vi "ex_FileReadTDM.vi"(0 "file path in":path, 1 "Read specified segment size":bool, 2 "First time?":bool, 3 "Ask user for file":bool, 4 "Segment Size":i32, 5 "error in (no error)":errorcluster, 6 "Plugin info":T1, 7 "read info in":T2, 9 "single values":bool, 10 "Lock file":bool) -> (13 "read info out":T2, 14 "file path out":path, 15 "Comment":string, 16 "Signals":waveform(dbl)[](array[waveform]), 17 "Description":string, 18 "EOF":bool, 19 "error out":errorcluster)   [LabVIEW 2020]
uses:
  <vilib>/Platform/express/TDMExpress.llb/ex_readInfoTDM.ctl
  <vilib>/Platform/express/TDMExpress.llb/ex_readChannelInfo.ctl
  <vilib>/express/express shared/ExFile.llb/ex_TdmData.ctl
  <vilib>/express/express shared/ExFile.llb/ex_TdmProperty.ctl
  <vilib>/express/express shared/ex_EditUserDefinedProperties/usiDataType.ctl
  <vilib>/express/express shared/ExFile.llb/ex_PluginInfo.ctl
  <vilib>/express/express shared/ExFile.llb/ex_FileFormatSelector.ctl
  <vilib>/express/express shared/ExFile.llb/ex_FileGlobals.vi
  <vilib>/Platform/storage/Storage.llb/__closeStorageFromObject.vi
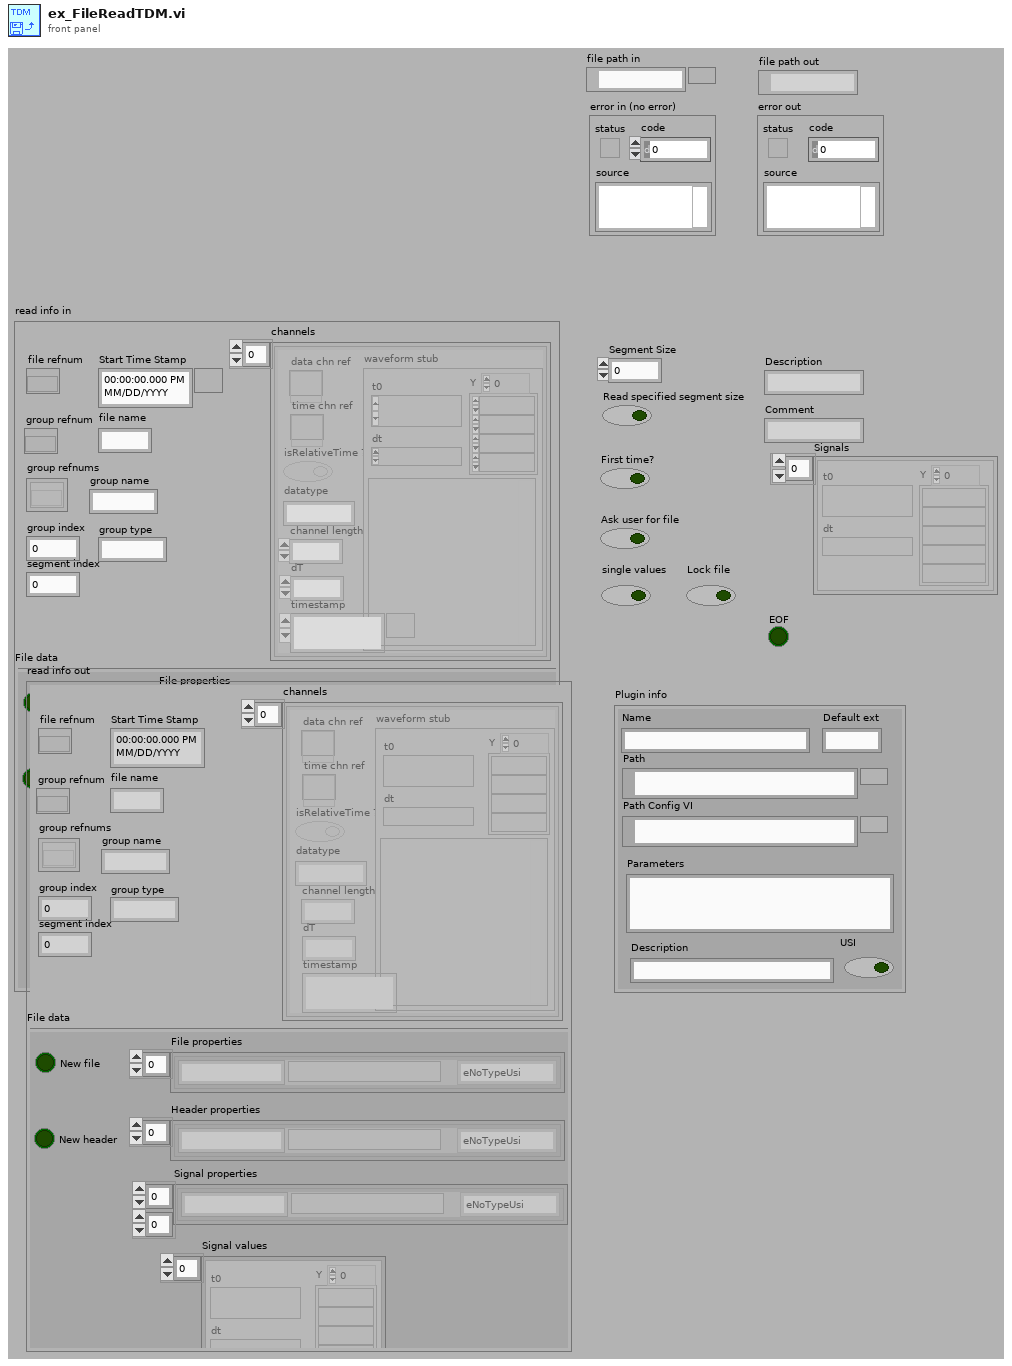
[diagram p1: front panel]
types:
  T1 = typedef "ex_PluginInfo.ctl" = cluster{"Name":string, "Path":path, "Default ext":string, "Parameters":string, "Path Config VI":path, "Description":string, "USI":bool}
  T2 = typedef "ex_readInfoTDM.ctl" = cluster{"file refnum":refnum<k20>, "group refnum":refnum<k20>, "group name":string, "group type":string, "Start Time Stamp":timestamp, "group index":u32, "group refnums":refnum<k20>[], "file name":string, "segment index":u32, "channels":T3[], "File data":T4}
  T3 = typedef "ex_readChannelInfo.ctl" = cluster{"data chn ref":refnum<k20>, "time chn ref":refnum<k20>, "isRelativeTime ?":bool, "channel length":u32, "dT":dbl, "waveform stub":waveform(dbl), "datatype":string, "timestamp":timestamp}
  T4 = typedef "ex_TdmData.ctl" = cluster{"New file":bool, "New header":bool, "File properties":T5[], "Header properties":T5[], "Signal properties":T5[][], "Signal values":waveform(dbl)[]}
  T5 = typedef "ex_TdmProperty.ctl" = cluster{"Name":string, "Type":T6, "Value":variant}
  T6 = typedef "usiDataType.ctl" = enum16{"eNoTypeUsi", "eInt8Usi", "eInt16Usi", "eInt32Usi", "eInt64Usi", "eUInt8Usi", "eUInt16Usi", "eUInt32Usi", "eUInt64Usi", "eFloat32Usi", "eFloat64Usi", "- 0", "- 1", "- 2", "- 3", "- 4", "- 5", "- 6", "- 7", "- 8", "- 9", "eString8Usi", "eString16Usi", "eStringUsi", "eEnumUsi", "- 10", "- 11", "- 12", "- 13", "- 14", "eTimeUsi", "- 15", "- 16", "- 17", "- 18", "- 19", "- 20", "- 21", "- 22", "- 23", "eInstanceUsi", "eStoreUsi"}
  T7 = typedef "ex_FileFormatSelector.ctl" = enum32{"lvm", "tdm", "other"}
  T8 = enum32{"existing file", "new file", "new or existing file", "existing dir", "new dir", "new or existing dir", "existing file (use LLBs)", "new file (use LLBs)", "new or existing file (use LLBs)", "new or existing file or directory (use LLBs)"}
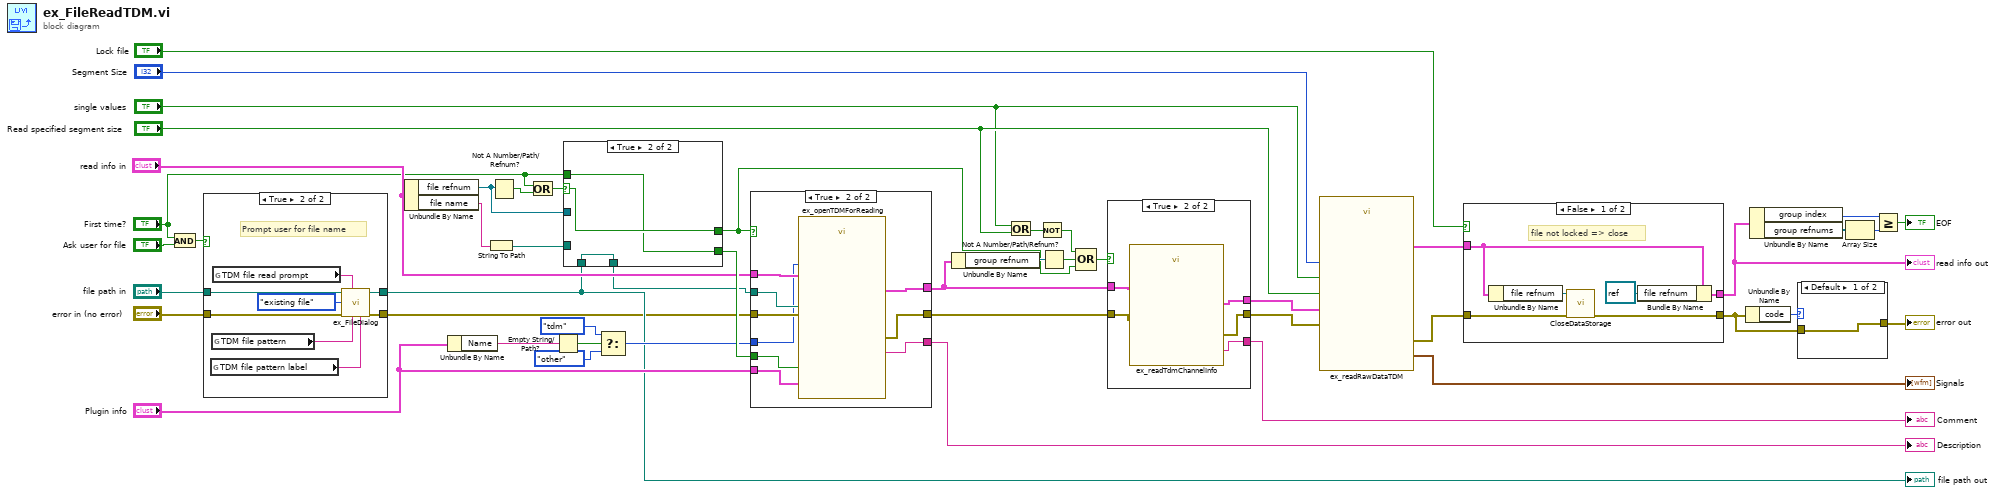
[diagram p0: block diagram]
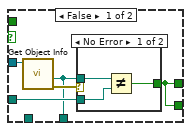
[diagram p2: hidden frame]
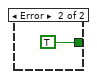
[diagram p3: hidden frame]
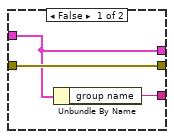
[diagram p4: hidden frame]
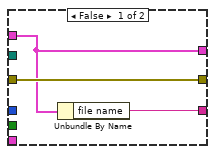
[diagram p6: hidden frame]
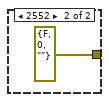
[diagram p7: hidden frame]
diagram:
  n1 = And(x="First time?", y="Ask user for file") -> (x .and. y?=w45:bool)
  n2 = case shown="True" w45 {
    tunnel: "file path in" -> [w50 w52]
    tunnel: [w49 w54] -> w1
    tunnel: [w50 w51] -> w6
    tunnel: "error in (no error)" -> [w49 w53]
    frame False {
      # "Use given file name"
    }
    frame True {
      # "Prompt user for file name"
      n3 = global read "ex_FileGlobals.vi" "TDM file pattern label"() -> (w55:string)
      n4 = global read "ex_FileGlobals.vi" "TDM file pattern"() -> (w56:string)
      n5 = global read "ex_FileGlobals.vi" "TDM file read prompt"() -> (w57:string)
      n6 = call <vilib>:"ex_FileDialog.vi"("pattern label"=w55, "pattern"=w56, "prompt"=w57, "error in (no error)"=w53, "select mode"=T8."existing file", "start path"=w52) -> ("error out"=w54:errorcluster, "selected file path"=w51:path)  [unwired: 4 out]
    }
  }
  "file path out" <- w6
  n7 = Unbundle By Name("read info in") -> ("file refnum"=w11:refnum<k20>, "file name"=w9:string)
  n8 = Unbundle By Name("Plugin info") -> ("Name"=w16:string)
  n9 = String To Path(string=w9) -> (path=w8:path)
  n10 = Not A Number/Path/Refnum?(number/path/refnum=w11) -> (NaN/Path/Refnum?=w5:bool)
  n11 = Or(x="First time?", y=w5) -> (x .or. y?=w3:bool)
  n12 = Empty String/Path?(string/path=w16) -> (empty?=w15:bool)
  n13 = case shown="True" w3 {
    selector: w3 -> [_ w70]
    tunnel: w11 -> [w63 _]
    tunnel: [w62 w70] -> w18
    tunnel: "First time?" -> [_ w69]
    tunnel: [w62 w69] -> w19
    tunnel: w8 -> [w60 _]
    tunnel: [w59 w68] -> w7
    tunnel: w6 -> [_ w68]
    frame False {
      n14 = call <vilib>:"Get Object Info.vi"("storage refnum"=w63) -> ("error out"=w61:errorcluster, "storage location"=w59:path)  [unwired: 1 in, 8 out]
      n15 = case shown="No Error" w61 {
        tunnel: w59 -> [w66 _]
        tunnel: [w65 TRUE] -> w62
        tunnel: w60 -> [w64 _]
        frame No Error {
          n16 = Not Equal?(x=w66, y=w64) -> (x != y?=w65:bool)
        }
        frame Error {
        }
      }
    }
    frame True {
    }
  }
  n17 = Select(t=ex_FileFormatSelector."tdm" ("storage_format"), s=w15, f=ex_FileFormatSelector."other" ("storage_format")) -> (s? t:f=w12:T7)
  n18 = case shown="True" w18 {
    tunnel: [w73 w81] -> w43
    tunnel: w1 -> [w73 w82]
    tunnel: w7 -> [_ w77]
    tunnel: "read info in" -> [w72 w80]
    tunnel: [w72 w79] -> w22
    tunnel: [w71 w78] -> w36
    tunnel: w19 -> [_ w76]
    tunnel: "Plugin info" -> [_ w75]
    tunnel: w12 -> [_ w74]
    frame False {
      n19 = Unbundle By Name(w72) -> ("file name"=w71:string)
    }
    frame True {
      n20 = call <vilib>:"ex_openTDMForReading.vi"("Plugin info"=w75, "storage_format"=w74, "error in (no error)"=w82, "read info  in"=w80, "Reset"=w76, "file path in"=w77) -> ("error out"=w81:errorcluster, "description"=w78:string, "read info  out"=w79:T2)  [unwired: 1 in, 2 out]
    }
  }
  "Description" <- w36
  n21 = Unbundle By Name(w22) -> ("group refnum"=w26:refnum<k20>)
  n22 = Or(x="single values", y="Read specified segment size") -> (x .or. y?=w25:bool)
  n23 = Not(x=w25) -> (.not. x?=w28:bool)
  n24 = Not A Number/Path/Refnum?(number/path/refnum=w26) -> (NaN/Path/Refnum?=w27:bool)
  n25 = Compound Arithmetic op=OR(w28, w27, w18) -> (w21:bool)
  n26 = case shown="True" w21 {
    tunnel: w43 -> [w85 w90]
    tunnel: [w85 w89] -> w39
    tunnel: [w83 w88] -> w35
    tunnel: [w84 w87] -> w2
    tunnel: w22 -> [w84 w86]
    frame False {
      n27 = Unbundle By Name(w84) -> ("group name"=w83:string)
    }
    frame True {
      n28 = call <vilib>:"ex_readTdmChannelInfo.vi"("error in (no error)"=w90, "read info in"=w86) -> ("error out"=w89:errorcluster, "read info out"=w87:T2, "comment"=w88:string)  [unwired: 2 in]
    }
  }
  "Comment" <- w35
  n29 = call <vilib>:"ex_readRawDataTDM.vi"("read info in"=w2, "single values"="single values", "specified size"="Read specified segment size", "segment size"="Segment Size", "error in (no error)"=w39) -> ("read info out"=w32:T2, "signals"=→"Signals":waveform(dbl)[], "error out"=w38:errorcluster)  [unwired: 5 in, 3 out]
  n30 = case shown="False" "Lock file" {
    tunnel: w38 -> [w96 w97]
    tunnel: [w95 w97] -> w37
    tunnel: w32 -> [w93 w98]
    tunnel: [w92 w98] -> w20
    frame False {
      # "file not locked => close"
      n31 = Unbundle By Name(w93) -> ("file refnum"=w94:refnum<k20>)
      n32 = call-poly <vilib>:"CloseDataStorage.vi"("error in (no error)"=w96, "storage refnum"=w94) -> ("error out"=w95:errorcluster)  [unwired: 5 out]
      n33 = Bundle By Name(cluster=w93, "file refnum"=refnum<k20> refnum) -> (w92:T2)
    }
    frame True {
    }
  }
  "read info out" <- w20
  n34 = Unbundle By Name(w37) -> ("code"=w42:i32)
  n35 = Unbundle By Name(w20) -> ("group index"=w31:u32, "group refnums"=w30:refnum<k20>[])
  n36 = case shown="Default" w42 {
    tunnel: w37 -> [w99 _]
    tunnel: [w99 errorcluster {"status"=FALSE, "code"=0, "source"=""} ("error out")] -> w41
    frame Default {
    }
    frame 2552 {
    }
  }
  "error out" <- w41
  n37 = Array Size(array=w30) -> (size(s)=w33:i32)
  n38 = Greater Or Equal?(x=w31, y=w33) -> (x >= y?=→"EOF":bool)
